vi "Dequeue Targets Update.vi"(0 "Targets Queue":refnum<queue>, 1 "error in":errorcluster) -> (2 "Targets Queue":refnum<queue>, 3 "Targets Update":T1, 4 "error out":errorcluster)   [LabVIEW 2016]
uses:
  Targets Update.ctl
  Targets Message.ctl
  Targets Info.ctl
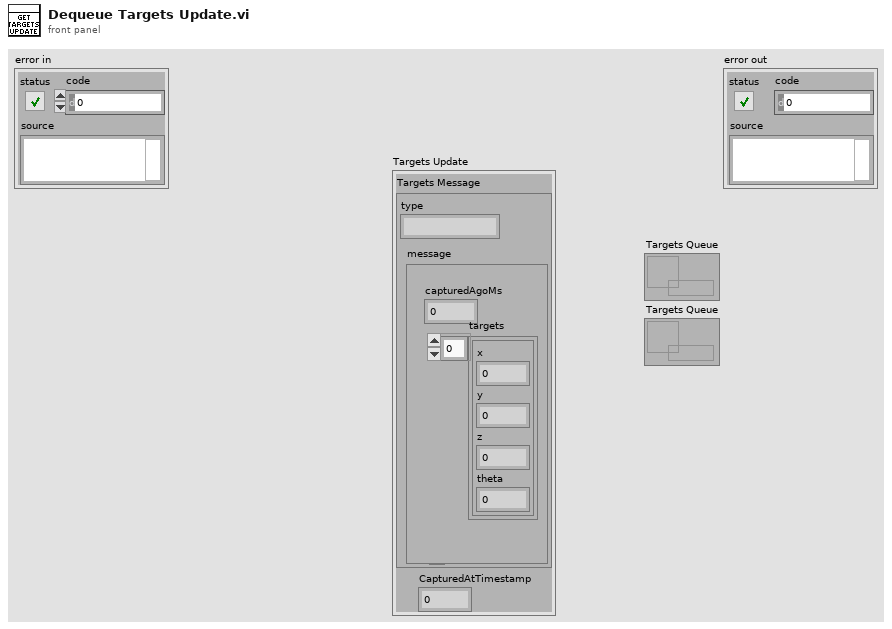
[diagram p1: front panel]
types:
  T1 = typedef "Targets Update.ctl" = cluster{"Valid?":bool, "CapturedAtTimestamp":dbl, "Targets Message":T2}
  T2 = typedef "Targets Message.ctl" = cluster{"type":string, "message":cluster{"capturedAgoMs":i32, "targets":T3[]}}
  T3 = typedef "Targets Info.ctl" = cluster{"x":dbl, "y":dbl, "z":dbl, "theta":dbl}
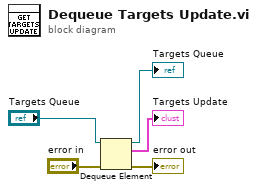
[diagram p0: block diagram]
diagram:
  n1 = Dequeue Element(queue="Targets Queue", error in (no error)="error in") -> (queue out=→"Targets Queue":refnum<queue>, element=→"Targets Update":T1, error out=→"error out":errorcluster)  [unwired: 1 in, 1 out]
